vi "RandomString.vi"() -> (2 "Random String":string)   [LabVIEW 2015, in "VIDiffUtilities.lvlib"]
uses:
  VIDiffUtilities.lvlib
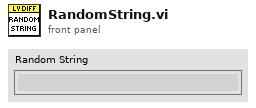
[diagram p1: front panel]
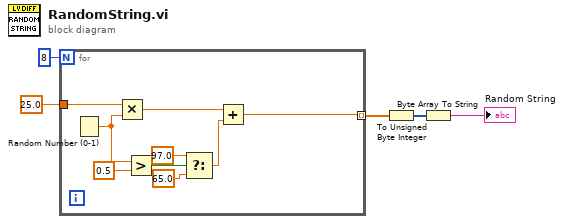
[diagram p0: block diagram]
diagram:
  n1 = for {
    N: 8 -> [_]
    tunnel: 25.0 -> [w13]
    tunnel: [w12] -> w3 mode=indexing
    n2 = Random Number (0-1)() -> (number: 0 to 1=w11:dbl)
    n3 = Multiply(x=w13, y=w11) -> (x*y=w14:dbl)
    n4 = Greater?(x=w11, y=0.5) -> (0:w9:bool)
    n5 = Select(t=97.0, s=w9, f=65.0) -> (s? t:f=w6:dbl)
    n6 = Add(x=w14, y=w6) -> (x+y=w12:dbl)
  }
  n7 = To Unsigned Byte Integer(number=w3) -> (unsigned 8bit integer=w2:u8[])
  n8 = Byte Array To String(unsigned byte array=w2) -> (string=→"Random String":string)
